vi "Get Velocity.vi"(8 "error in (no error)":errorcluster, 11 "ODESimulator_Base_Conveyor in":refnum<class "ODESimulator_Base_Conveyor.lvclass">) -> (0 "error out":errorcluster, 2 "Velocity":dbl, 3 "ODESimulator_Base_Conveyor out":refnum<class "ODESimulator_Base_Conveyor.lvclass">)   [LabVIEW 2017, in "NI_Robotics_Simulator.lvlib" / "ODESimulator_Base_Conveyor.lvclass"]
uses:
  <vilib>/robotics/Simulator/Robot Factory/Conveyor/Base/ODESimulator_Base_Conveyor.lvclass
  <vilib>/robotics/Simulator/Robot Factory/Conveyor/Base/ODESimulator_Base_Conveyor.lvclass/ODESimulator_Base_Conveyor.ctl
  <resource>/objmgr/LVODE.rc
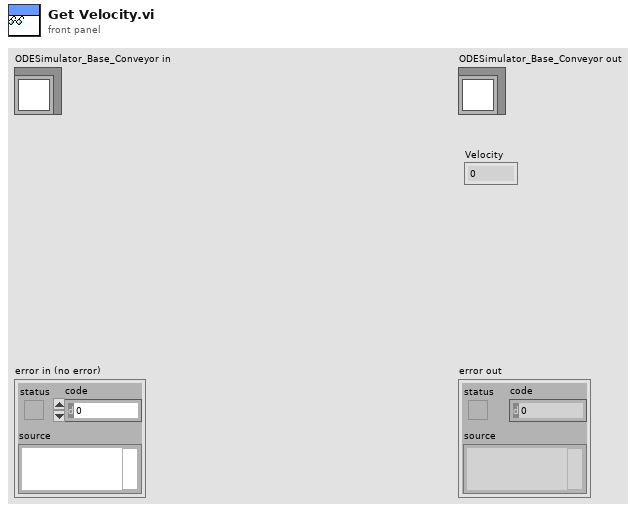
[diagram p1: front panel]
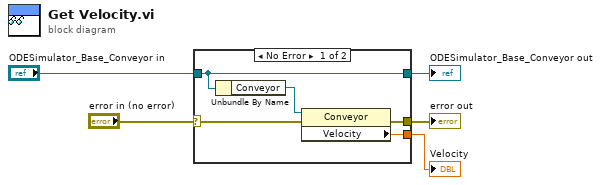
[diagram p0: block diagram]
diagram:
  n1 = case shown="No Error" "error in (no error)" {
    selector: "error in (no error)" -> [w7 w11]
    tunnel: [w6 w11] -> w4
    tunnel: [w10 w12] -> w2
    tunnel: "ODESimulator_Base_Conveyor in" -> [w10 w12]
    tunnel: [w8 _] -> w1
    frame No Error {
      n2 = Unbundle By Name(w10) -> ("Conveyor"=w9:refnum<k20>)
      n3 = property class="Conveyor"(reference=w9, error in=w7) -> (error out=w6:errorcluster, "Velocity"=w8:sgl)  [unwired: 1 out]
    }
    frame Error {
    }
  }
  "error out" <- w4
  "ODESimulator_Base_Conveyor out" <- w2
  "Velocity" <- w1
